vi "Read motor by name.vi"(8 "error in (no error)":errorcluster, 10 "motor name":string, 11 "ICS in":refnum<class "ICS.lvclass">) -> (0 "error out":errorcluster, 1 "index":i32, 2 "Motor.lvclass":refnum<class "Motor.lvclass">, 3 "ICS out":refnum<class "ICS.lvclass">)   [LabVIEW 2018, in "ICS.lvclass"]
uses:
  ICS.lvclass
  Motor/Motor.lvclass
  ICS.lvclass/ICS.ctl
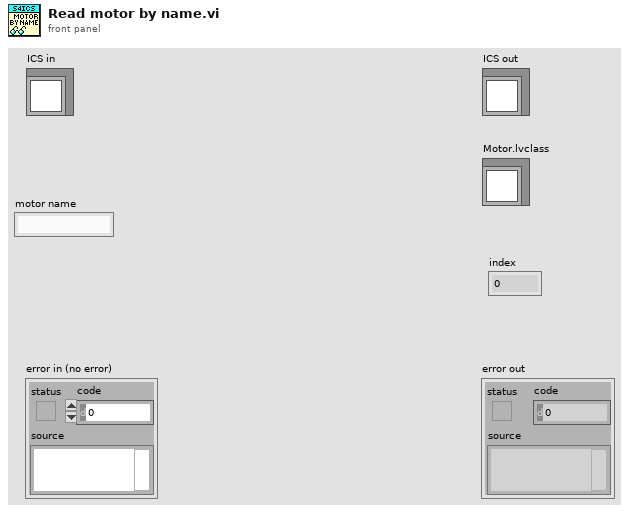
[diagram p1: front panel]
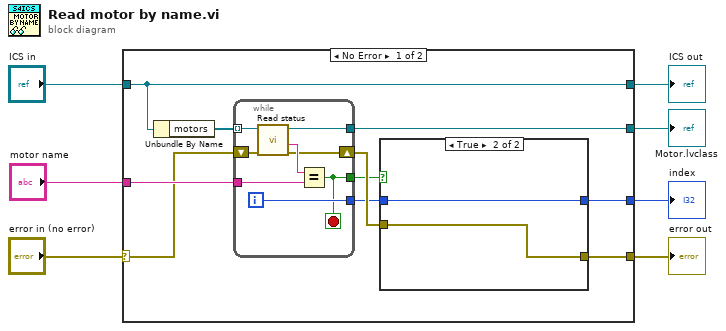
[diagram p0: block diagram]
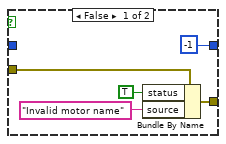
[diagram p2: hidden frame]
diagram:
  n1 = case shown="No Error" "error in (no error)" {
    selector: "error in (no error)" -> [w13 w33]
    tunnel: [w11 w33] -> w6
    tunnel: [w17 w34] -> w4
    tunnel: "ICS in" -> [w17 w34]
    tunnel: [w15 _] -> w3
    tunnel: "motor name" -> [w16 _]
    tunnel: [w9 _] -> w1
    frame No Error {
      n2 = Unbundle By Name(w17) -> ("motors"=w14:refnum<class "Motor.lvclass">[])
      n3 = while {
        tunnel: w14 -> [w25] mode=indexing
        tunnel: w16 -> [w22]
        tunnel: [w21] -> w15
        shift-right: [w20] -> w12
        shift-left: w13 -> [w24]
        tunnel: [w19] -> w10
        tunnel: [w18] -> w8
        i -> [w19]
        stop <- w18 stop-if-true
        n4 = call-dynamic "Read status.vi"("error in (no error)"=w24, "Motor in"=w25) -> ("error out"=w20:errorcluster, "name"=w23:string, "Motor out"=w21:refnum<class "Motor.lvclass">)  [unwired: 6 in, 1 out]
        n5 = Equal?(x=w23, y=w22) -> (x = y?=w18:bool)
      }
      n6 = case shown="True" w8 {
        tunnel: w12 -> [w30 w32]
        tunnel: [w29 w32] -> w11
        tunnel: w10 -> [_ w31]
        tunnel: [-1 w31] -> w9
        frame False {
          n7 = Bundle By Name(cluster=w30, "status"=TRUE, "source"="Invalid motor name") -> (w29:errorcluster)
        }
        frame True {
        }
      }
    }
    frame Error {
    }
  }
  "error out" <- w6
  "ICS out" <- w4
  "Motor.lvclass" <- w3
  "index" <- w1
